vi "0254-write-reference.vi"(9 "SV":dbl, 10 "Channel Selection":i32, 11 "VISA Refnum in":refnum<visa-resource-name>) -> (0 "error out":errorcluster, 2 "SV_CH1":dbl, 3 "VISA Refnum out":refnum<visa-resource-name>)   [LabVIEW 2015]
uses:
  <vilib>/Instr/_visa.llb/VISA Configure Serial Port (Instr).vi
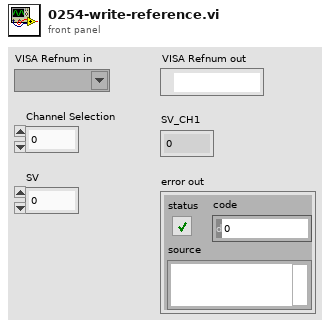
[diagram p1: front panel]
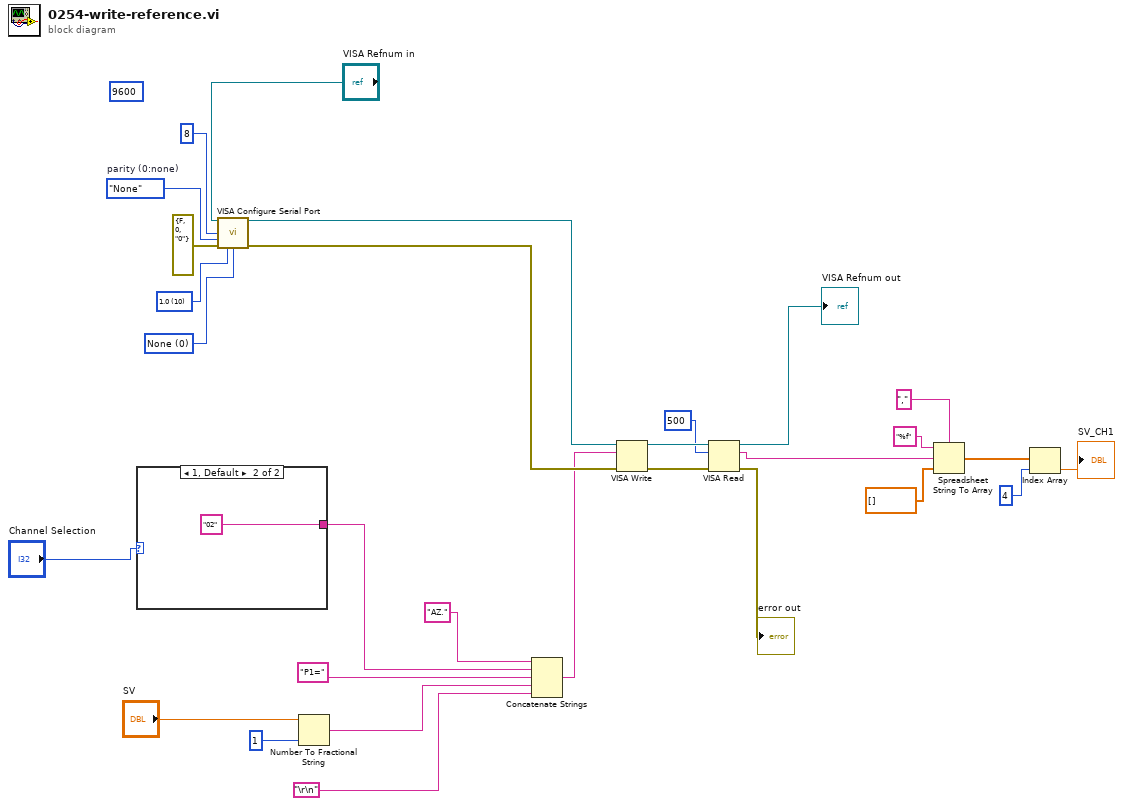
[diagram p0: block diagram]
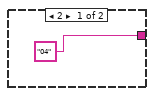
[diagram p2: hidden frame]
diagram:
  w17 = u16 0 items=["None", "XON/XOFF", "RTS/CTS", "XON/XOFF & RTS/CTS", "DTR/DSR", "XON/XOFF & DTR/DSR"] ("flow control (0:none)")
  w16 = u16 10 items=["1.0"=10, "1.5"=15, "2.0"=20] ("stop bits (10: 1 bit)")
  w15 = enum16{"None", "Odd", "Even", "Mark", "Space"}."None"  # parity (0:none)
  (unwired) u32 9600 ("baud rate (9600)")
  n1 = case shown="1, Default" "Channel Selection" {
    tunnel: ["04" "02"] -> w25
    frame 2 {
    }
    frame 1, Default {
    }
  }
  n2 = call-poly "VISA Configure Serial Port"("VISA resource name"="VISA Refnum in", "data bits (8)"=u16 8, "parity (0:none)"=w15, "error in (no error)"=errorcluster {"status"=FALSE, "code"=0, "source"="0"}, "stop bits (10: 1 bit)"=w16, "flow control (0:none)"=w17) -> ("VISA resource name out"=w21:refnum<visa-resource-name>, "error out"=w22:errorcluster)  [unwired: 8 in]
  n3 = Number To Fractional String(number="SV", precision (6)=i16 1) -> (F-format string=w23:string)  [unwired: 2 in]
  n4 = Concatenate Strings("AZ." ("string"), w25, "P1=" ("string"), w23, "\r\n") -> (w5:string)
  n5 = VISA Write(VISA resource name=w21, write buffer=w5, error in (no error)=w22) -> (VISA resource name out=w4:refnum<visa-resource-name>, error out=w2:errorcluster)  [unwired: 1 out]
  n6 = VISA Read(VISA resource name=w4, byte count=u32 500, error in (no error)=w2) -> (VISA resource name out=→"VISA Refnum out":refnum<visa-resource-name>, read buffer=w10:string, error out=→"error out":errorcluster)  [unwired: 1 out]
  n7 = Spreadsheet String To Array(delimiter (Tab)=",", format string="%f", spreadsheet string=w10, array type (2D Dbl)=dbl[] []) -> (array=w7:dbl[])
  n8 = Index Array(array=w7, index=4) -> (element=→"SV_CH1":dbl)
